vi "Transfer Teleop.vi"() -> ()   [LabVIEW 2020]
panel:
  in  "Conveyer 2":dbl
  in  "Conveyer 1":dbl
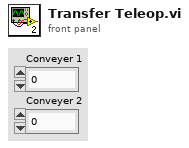
[diagram p1: front panel]
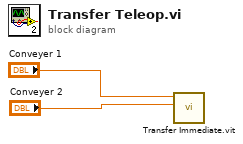
[diagram p0: block diagram]
diagram:
  n1 = call "Transfer Immediate.vit"("Conveyer 2"="Conveyer 2", "Conveyer 1"="Conveyer 1") -> ()  [unwired: 9 in, 1 out]
